vi "UpdateStateMax&Min.vi"(10 "ControlState":T2(ring), 11 "Array in":cluster{"SensorCluster":T1}[](array[cluster])) -> (3 "Array out":cluster{"SensorCluster":T1}[](array[cluster]))   [LabVIEW 2018]
uses:
  Type_Def ClusterSensor.ctl
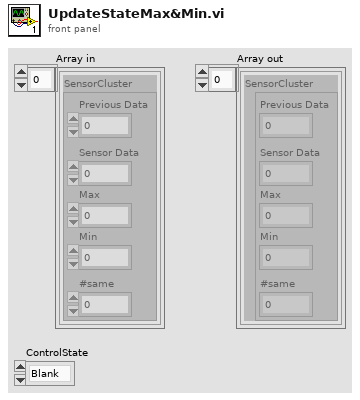
[diagram p1: front panel]
types:
  T1 = typedef "Type_Def ClusterSensor.ctl" = cluster{"Sensor Data":dbl, "Max":dbl, "Min":dbl, "Previous Data":dbl, "#same":dbl}
  T2 = enum16{"Blank", "Systems Check", "Idle", "Ready", "Pushing", "CrawlingPrecharge", "Braking", "Fault", "Boot Up", "Unpowered", "Crawling", "Shutdown", "Service Push", "Service Wait", "Vent", "Precharge", "Cooldown"}
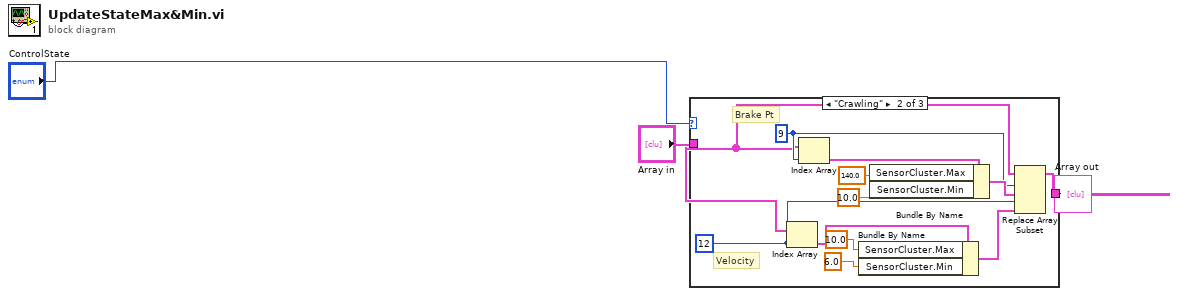
[diagram p0: block diagram]
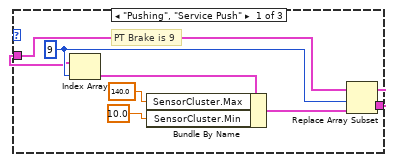
[diagram p2: hidden frame]
diagram:
  n1 = case shown="\"Crawling\"" "ControlState" {
    tunnel: [w10 w22 w23] -> w1
    tunnel: "Array in" -> [w4 w11 w23]
    frame "Pushing", "Service Push" {
      w6 = 9 ("index")
      # "PT Brake is 9"
      n2 = Index Array(array=w4, index=w6) -> (element=w5:cluster{"SensorCluster":T1})
      n3 = Bundle By Name(cluster=w5, "SensorCluster.Max"=140.0, "SensorCluster.Min"=10.0) -> (w7:cluster{"SensorCluster":T1})
      n4 = Replace Array Subset(array=w4, new element=w7, index=w6) -> (w10:cluster{"SensorCluster":T1}[])
    }
    frame "Crawling" {
      w14 = 12 ("index")
      w18 = 9 ("index")
      # "Velocity"
      # "Brake Pt"
      n5 = Index Array(array=w11, index=w14) -> (element=w12:cluster{"SensorCluster":T1})
      n6 = Index Array(array=w11, index=w18) -> (element=w13:cluster{"SensorCluster":T1})
      n7 = Bundle By Name(cluster=w12, "SensorCluster.Max"=10.0, "SensorCluster.Min"=6.0) -> (w15:cluster{"SensorCluster":T1})
      n8 = Bundle By Name(cluster=w13, "SensorCluster.Max"=140.0, "SensorCluster.Min"=10.0) -> (w19:cluster{"SensorCluster":T1})
      n9 = Replace Array Subset(array=w11, new element #1=w19, index #1=w18, new element #2=w15, index #2=w14) -> (w22:cluster{"SensorCluster":T1}[])
    }
    frame Default {
    }
  }
  "Array out" <- w1
